vi "Create Evaluations.vi"(8 "error in (no error)":errorcluster, 11 "IEvaluation in":refnum<class "CDMA2K_ACP.lvclass">) -> (0 "error out":errorcluster, 2 "Evaluations Out":T1[](array[typedef]) {"Low Limit" format="%#_13g"; "SI Scaling" items=["femto"=-15, "pico"=-12, "nano"=-9, "micro"=-6, "milli"=-3, "percent"=-2, ""=0, "kilo"=3, "mega"=6, "giga"=9, "tera"=12]}, 3 "IEvaluation out":refnum<class "CDMA2K_ACP.lvclass">)   [LabVIEW 2016, in "SeqAuto Evaluations.lvlib" / "CDMA2K_ACP.lvclass"]
uses:
  CDMA2K_ACP.lvclass
  C:/projects/STS/Common/Sequence Automation/Plugins/SeqAuto IEvaluation.lvlibp/SeqAuto IEvaluation.lvclass
  Plugins/TestStand API Tools (TSAT).lvlibp/Evaluation Actions/Includes/Controls/TSAT Evaluation.ctl
  Plugins/TestStand API Tools (TSAT).lvlibp/Evaluation Actions/Includes/Controls/TSAT Eval SI Unit Scaling.ctl
  Plugins/TestStand API Tools (TSAT).lvlibp/Evaluation Actions/Includes/Controls/TSAT Evaluation Type.ctl
  Plugins/SeqAuto IEvaluation.lvlibp/Read Measurement Name.vi
  Plugins/TestStand API Tools (TSAT).lvlibp/Evaluation Actions/TSAT Evaluation Actions.lvlib
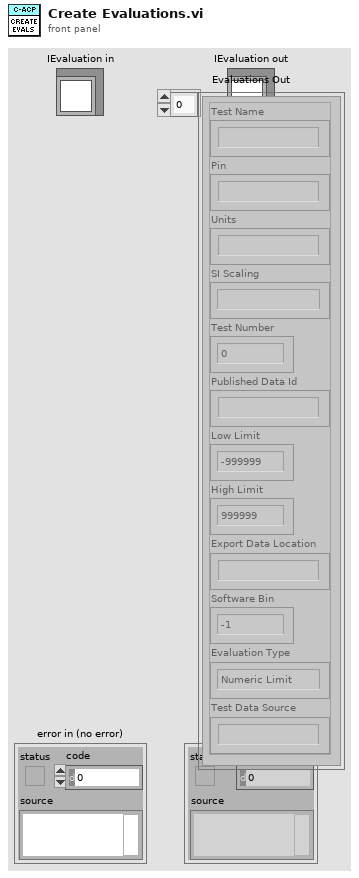
[diagram p1: front panel]
types:
  T1 = typedef "TestStand API Tools (TSAT).lvlibp/TSAT Evaluation Actions.lvlib/TSAT Evaluation.ctl" = cluster{"Test Name":string, "Pin":string, "Units":string, "SI Scaling":T2, "Test Number":i32, "Published Data Id":string, "Low Limit":dbl, "High Limit":dbl, "Export Data Location":string, "Software Bin":i64, "Evaluation Type":T3, "Test Data Source":string}
  T2 = typedef "TestStand API Tools (TSAT).lvlibp/TSAT Evaluation Actions.lvlib/TSAT Eval SI Unit Scaling.ctl" = i16
  T3 = typedef "TestStand API Tools (TSAT).lvlibp/TSAT Evaluation Actions.lvlib/TSAT Evaluation Type.ctl" = enum16{"Numeric Limit", "Pass/Fail", "None"}
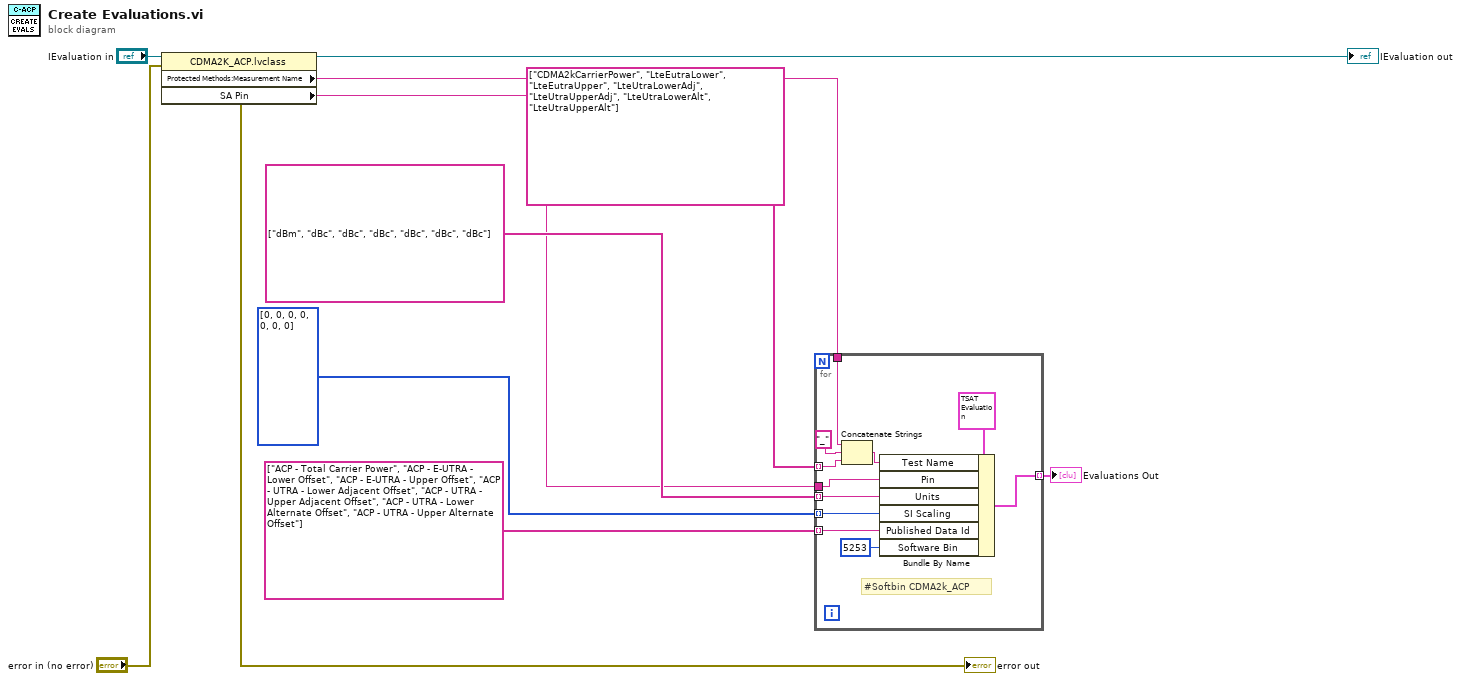
[diagram p0: block diagram]
diagram:
  w6 = T2[] [0, 0, 0, 0, 0, 0, 0] items=["femto"=-15, "pico"=-12, "nano"=-9, "micro"=-6, "milli"=-3, "percent"=-2, ""=0, "kilo"=3, "mega"=6, "giga"=9, "tera"=12]
  n1 = property class="CDMA2K_ACP.lvclass"(reference="IEvaluation in", error in="error in (no error)") -> (reference out=→"IEvaluation out":refnum<class "CDMA2K_ACP.lvclass">, error out=→"error out":errorcluster, "Protected Methods:Measurement Name"=w4:string, "SA Pin"=w2:string)
  n2 = for {
    tunnel: [w21] -> w1 mode=indexing
    tunnel: string[] ["ACP - Total Carrier Power", "ACP - E-UTRA - Lower Offset", "ACP - E-UTRA - Upper Offset", "ACP - UTRA - Lower Adjacent Offset", "ACP - UTRA - Upper Adjacent Offset", "ACP - UTRA - Lower Alternate Offset", "ACP - UTRA - Upper Alternate Offset"] ("Array") -> [w20] mode=indexing
    tunnel: w6 -> [w19] mode=indexing
    tunnel: string[] ["dBm", "dBc", "dBc", "dBc", "dBc", "dBc", "dBc"] ("Array") -> [w18] mode=indexing
    tunnel: w4 -> [w15]
    tunnel: string[] ["CDMA2kCarrierPower", "LteEutraLower", "LteEutraUpper", "LteUtraLowerAdj", "LteUtraUpperAdj", "LteUtraLowerAlt", "LteUtraUpperAlt"] -> [w14] mode=indexing
    tunnel: w2 -> [w13]
    # "#Softbin CDMA2k_ACP"
    n3 = Concatenate Strings(w15, "_" ("string"), w14) -> (w17:string)
    n4 = Bundle By Name(cluster=T1 {"Test Name"="", "Pin"="", "Units"="", "SI Scaling"=0, "Test Number"=0, "Published Data Id"="", "Low Limit"=-999999.0, "High Limit"=999999.0, "Export Data Location"="", "Software Bin"=-1, "Evaluation Type"=enum."Numeric Limit", "Test Data Source"=""} ("Evaluation"), "Test Name"=w17, "Pin"=w13, "Units"=w18, "SI Scaling"=w19, "Published Data Id"=w20, "Software Bin"=i64 5253) -> (w21:T1)
  }
  "Evaluations Out" <- w1
